vi "calibrateWavelength.vi"(8 "error in (no error)":errorcluster, 9 "Monochromator in":refnum<class "Monochromator.lvclass">, 10 "wavelength":T1, 11 "ReadySate in":refnum<class "ReadySate.lvclass">) -> (0 "error out":errorcluster, 1 "Monochromator out":refnum<class "Monochromator.lvclass">, 3 "ReadySate out":refnum<class "ReadySate.lvclass">)   [LabVIEW 2016, in "ReadySate.lvclass"]
uses:
  ReadySate.lvclass
  Typedefs/wavelength.ctl
  Monochromator/Monochromator.lvclass
  Typedefs/SWStatus.ctl
  Typedefs/AckType.ctl
  Monochromator/Monochromator.lvclass/Monochromator.ctl
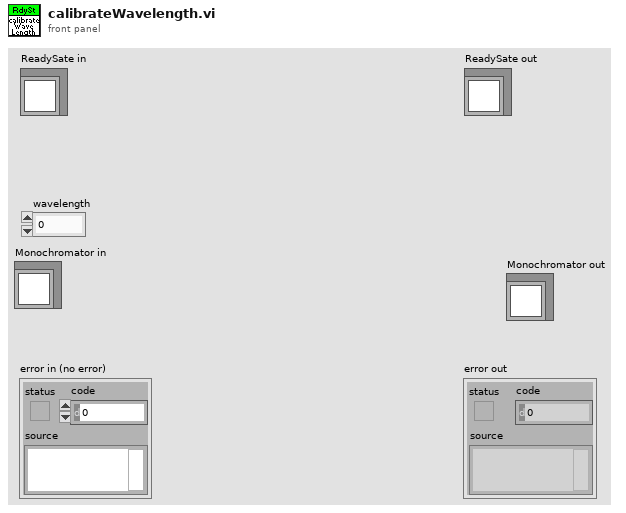
[diagram p1: front panel]
types:
  T1 = typedef "wavelength.ctl" = dbl
  T2 = typedef "AckType.ctl" = enum16{"OK", "OutOfRange", "Unknown", "Busy", "Rejected"}
  T3 = typedef "SWStatus.ctl" = enum16{"OfflineState", "ReadyState", "SettingUpState", "FaultState"}
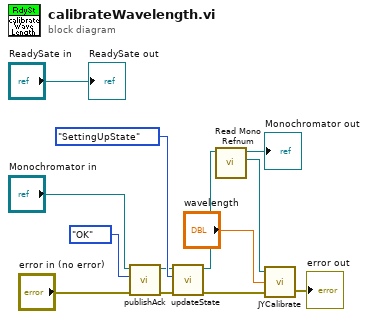
[diagram p0: block diagram]
diagram:
  n1 = call "publishAck.vi"("error in (no error)"="error in (no error)", "Ack"=AckType."OK" ("AckType"), "Monochromator in"="Monochromator in") -> ("error out"=w10:errorcluster, "Monochromator out"=w9:refnum<class "Monochromator.lvclass">)  [unwired: 7 in]
  n2 = call "updateState.vi"("error in (no error)"=w10, "SWStatus"=SWStatus."SettingUpState", "Monochromator in"=w9) -> ("error out"=w3:errorcluster, "Monochromator out"=w6:refnum<class "Monochromator.lvclass">)  [unwired: 7 in]
  n3 = call "Read Mono Refnum.vi"("Monochromator in"=w6) -> ("Mono Refnum"=w1:refnum<k7>, "Monochromator out"=→"Monochromator out":refnum<class "Monochromator.lvclass">)  [unwired: 8 in, 1 out]
  n4 = call "JYCalibrate.vi"("error in (no error)"=w3, "Actual Wavelength"="wavelength", "JYMONOLib.IJYMonoReqd"=w1) -> ("error out"=→"error out":errorcluster)  [unwired: 1 out]
  "ReadySate out" <- "ReadySate in"
